vi "Set ThrowAway.vi"(8 "error in (no error)":errorcluster, 10 "ThrowAway (0)":i32=1 min=0 max=2000 step=1, 11 "VISA resource name":refnum<visa-resource-name>) -> (0 "error out":errorcluster, 3 "VISA resource name out":refnum<visa-resource-name>)   [LabVIEW 2025, in "Detector SCPI.lvlib"]
doc: "Sets number of readings to discard at the start of each burst"
uses:
  Detector SCPI.lvlib
panel:
  out "Error Message":string
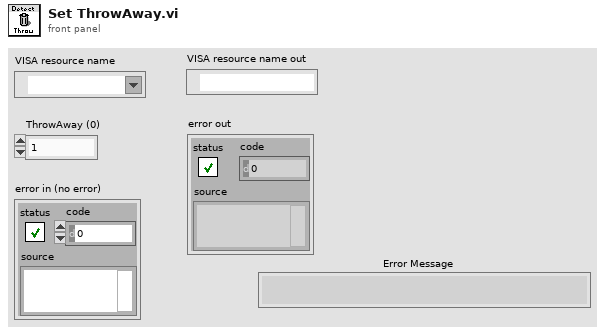
[diagram p1: front panel]
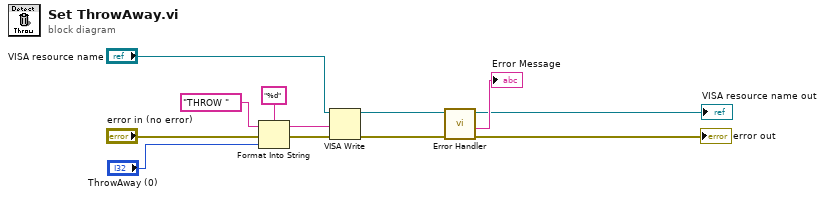
[diagram p0: block diagram]
diagram:
  n1 = Format Into String(format string="%d", initial string="THROW " ("command"), error in="error in (no error)", "ThrowAway (0)") -> (resulting string=w6:string, error out=w10:errorcluster)
  n2 = VISA Write(VISA resource name="VISA resource name", write buffer=w6, error in (no error)=w10) -> (VISA resource name out=w4:refnum<visa-resource-name>, error out=w3:errorcluster)  [unwired: 1 out]
  n3 = call "Error Handler.vi"("error in (no error)"=w3, "VISA resource name"=w4) -> ("error out"=→"error out":errorcluster, "Error Message"=→"Error Message":string, "VISA resource name out"=→"VISA resource name out":refnum<visa-resource-name>)  [unwired: 7 in]
